vi "readAppConfigFile.vi"(8 "Error In":errorcluster, 11 "App Config File Path":path) -> (0 "Error Out":errorcluster, 1 "isSimulation?":bool, 2 "Software Name":string, 3 "Company Name":string)   [LabVIEW 2018]
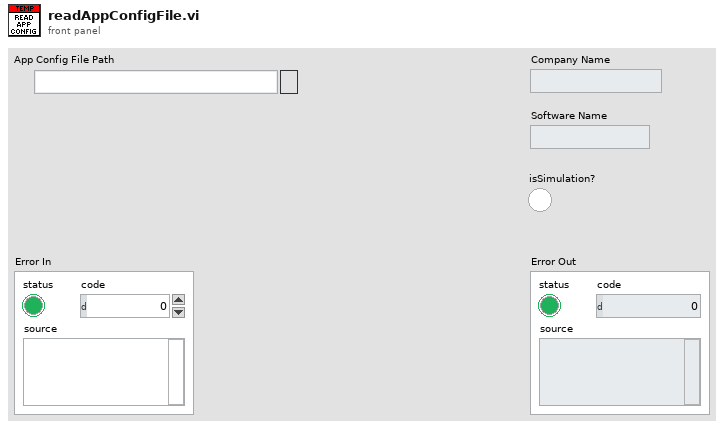
[diagram p1: front panel]
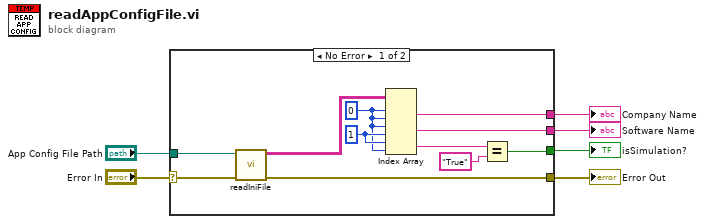
[diagram p0: block diagram]
diagram:
  n1 = case shown="No Error" "Error In" {
    selector: "Error In" -> [w17 w18]
    tunnel: [w16 w18] -> w5
    tunnel: "App Config File Path" -> [w15 _]
    tunnel: [w11 _] -> w3
    tunnel: [w10 _] -> w2
    tunnel: [w7 _] -> w1
    frame No Error {
      w13 = 1 ("index (row)")
      w12 = 0 ("index (row)")
      n2 = call "readIniFile.vi"("Error In"=w17, "File Path Control"=w15) -> ("Error Out"=w16:errorcluster, "Value"=w14:string[][])  [unwired: 8 in]
      n3 = Index Array(array=w14, index (row) #1=w12, index (col) #1=w12, index (row) #2=w12, index (col) #2=w13, index (row) #3=w13, index (col) #3=w12) -> (element #1=w11:string, element #2=w10:string, element #3=w9:string)
      n4 = Equal?(x=w9, y="True") -> (x = y?=w7:bool)
    }
    frame Error {
    }
  }
  "Error Out" <- w5
  "Company Name" <- w3
  "Software Name" <- w2
  "isSimulation?" <- w1
